vi "createDict.vi"(8 "error in (no error)":errorcluster) -> (0 "error out":errorcluster, 3 "IDict out":refnum<class "IDict.lvclass">)   [LabVIEW 2022 SP3, in "openDAQ.lvlib" / "daqCoreTypes.lvlib" / "IDict.lvclass"]
uses:
  <instrlib>/openDAQ/Public/Classes/daqCoreTypes/IDict/IDict.lvclass
  <instrlib>/openDAQ/Public/Classes/daqCoreTypes/IDict/IDict.lvclass/IDict.ctl
  <instrlib>/openDAQ/Binaries/Windows/x86/copendaq32.dll
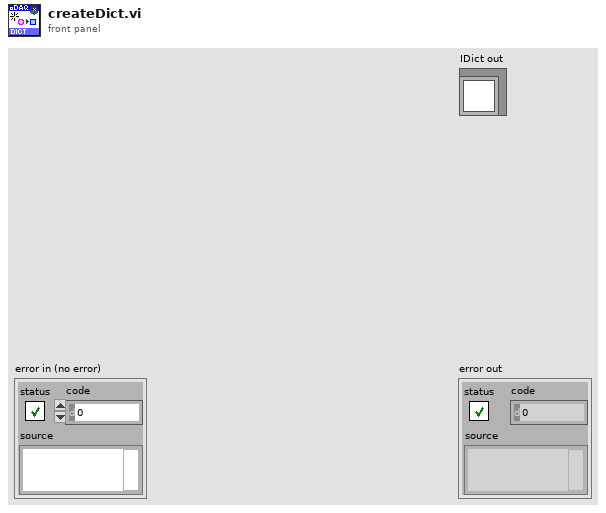
[diagram p1: front panel]
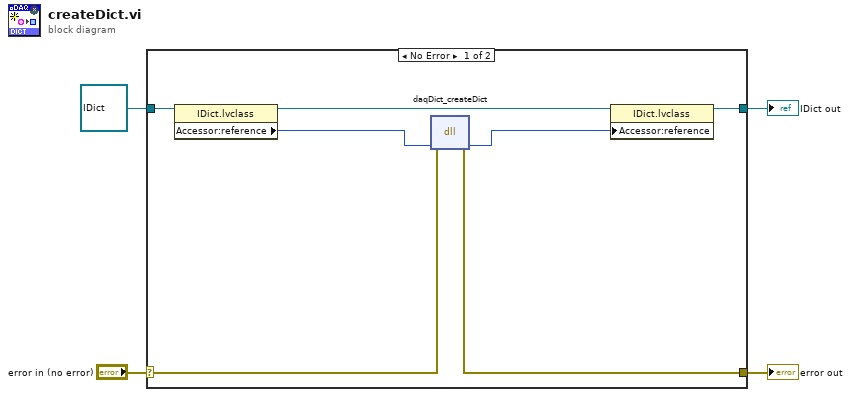
[diagram p0: block diagram]
diagram:
  n1 = case shown="No Error" "error in (no error)" {
    selector: "error in (no error)" -> [w6 w13]
    tunnel: [w5 w13] -> w3
    tunnel: [w8 w12] -> w1
    tunnel: refnum<class "IDict.lvclass"> refnum ("IDict in") -> [w11 w12]
    frame No Error {
      n2 = property class="IDict.lvclass"(reference=w11) -> (reference out=w9:refnum<class "IDict.lvclass">, "Accessor:reference"=w10:i64)  [unwired: 1 in, 1 out]
      n3 = dll-call lib="C:/Program Files (x86)/National Instruments/LabVIEW 2022/instr.lib/openDAQ/Binaries/Windows/x86/copendaq*.*" fn="daqDict_createDict"(error in=w6, "dict"=w10) -> (error out=w5:errorcluster, "dict"=w7:i64)  [unwired: 3 in, 1 out]
      n4 = property class="IDict.lvclass"(reference=w9, "Accessor:reference"=w7) -> (reference out=w8:refnum<class "IDict.lvclass">)  [unwired: 1 in, 1 out]
    }
    frame Error {
    }
  }
  "error out" <- w3
  "IDict out" <- w1
